vi "Self Test.vi"(8 "error in (no error)":errorcluster, 11 "Instruments in":refnum<class "Instruments.lvclass">) -> (0 "error out":errorcluster, 3 "Instruments out":refnum<class "Instruments.lvclass">)   [LabVIEW 2023, in "Instruments.lvlib" / "Instruments.lvclass"]
doc: "<b>Self Test</b>\n\nDescendents must override this routine\n\nSelf test is meant to check the health of an instrument after the device has been connected. \nThis routine is called in the Instrument Class Connect routine"
uses:
  Library/Instruments.lvclass
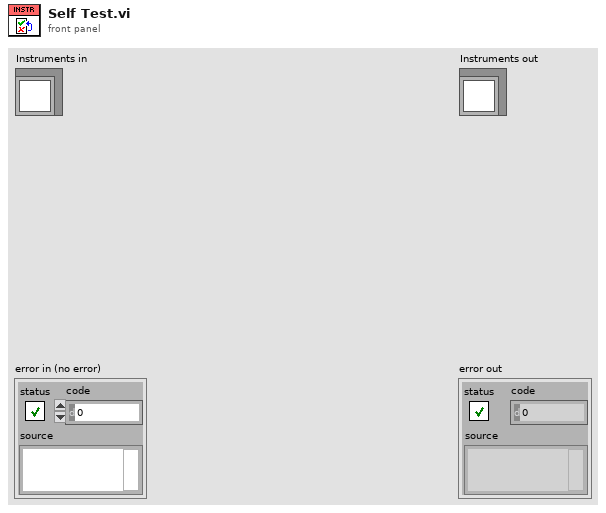
[diagram p1: front panel]
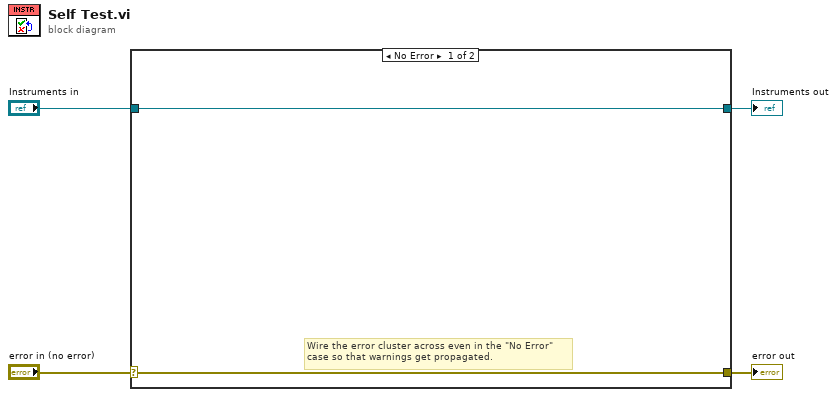
[diagram p0: block diagram]
diagram:
  n1 = case shown="No Error" "error in (no error)" {
    selector: "error in (no error)" -> [w5 w8]
    tunnel: [w5 w8] -> w3
    tunnel: [w6 w7] -> w1
    tunnel: "Instruments in" -> [w6 w7]
    frame No Error {
      # "Wire the error cluster across even in the \"No Error\"\ncase so that warnings get propagated."
    }
    frame Error {
    }
  }
  "error out" <- w3
  "Instruments out" <- w1
